vi "DBL Variant or Array Variant to Array.vi"(8 "error in (no error)":errorcluster, 11 "value":variant) -> (0 "error out":errorcluster, 3 "Array":dbl[](array[numeric]))   [LabVIEW 2019, in "SMO.Control Experiment.lvclass"]
uses:
  SMO.Control Experiment.lvclass
  <vilib>/Utility/Data Type/NI_Data Type.lvlib
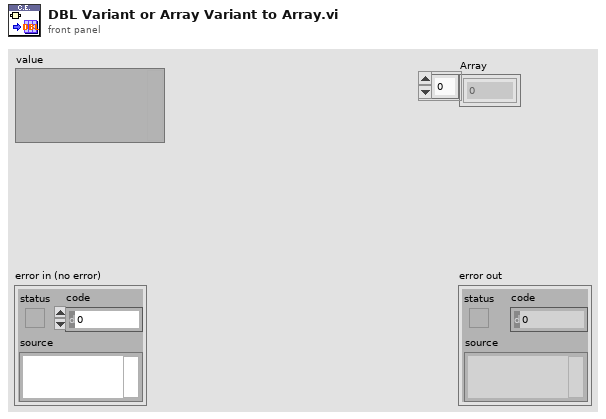
[diagram p1: front panel]
types:
  T1 = typedef "NI_Data Type.lvlib/Data Type.ctl" = enum8{"Invalid Type", "Void", "I8", "I16", "I32", "I64", "U8", "U16", "U32", "U64", "Single Float", "Double Float", "Extended Float", "Single Complex", "Double Complex", "Extended Complex", "Enum U8", "Enum U16", "Enum U32", "Enum U64", "Single Float With Unit", "Double Float With Unit", "Extended Float With Unit", "Single Complex with Unit", "Double Complex with Unit", "Extended Complex with Unit", "Boolean", "String", "Path", "Picture", "Tag", "Array", "Cluster", "Variant", "LV Variant", "Waveform", "Timestamp", "Digital Waveform", "Digital Data", "ExpressData", "Refnum", "External Data", "VI", "Poly VI", "LabVIEW Class Instance", "Fixed Point", "Set Collection", "Map Collection"}
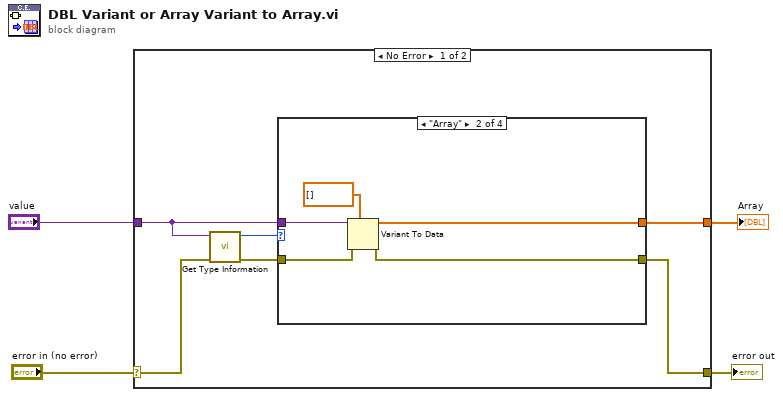
[diagram p0: block diagram]
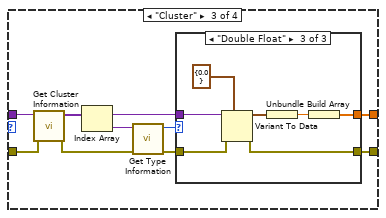
[diagram p3: hidden frame]
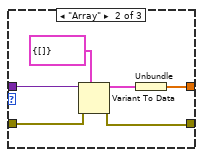
[diagram p5: hidden frame]
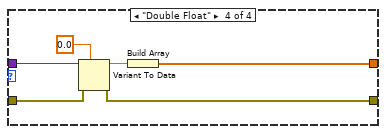
[diagram p6: hidden frame]
diagram:
  n1 = case shown="No Error" "error in (no error)" {
    selector: "error in (no error)" -> [w8 w46]
    tunnel: [w5 w46] -> w3
    tunnel: "value" -> [w9 _]
    tunnel: [w7 _] -> w1
    frame No Error {
      n2 = call <vilib>:"Get Type Information.vi"("error in (no error)"=w8, "variant"=w9) -> ("error out"=w6:errorcluster, "type"=w10:T1)  [unwired: 5 in, 3 out]
      n3 = case shown="\"Array\"" w10 {
        tunnel: [_ w15 w19 w41] -> w7
        tunnel: w9 -> [_ w14 w17 w44]
        tunnel: w6 -> [w11 w13 w25 w43]
        tunnel: [w11 w12 w18 w40] -> w5
        frame Default {
        }
        frame "Array" {
          n4 = Variant To Data(error in=w13, type=dbl[] [], Variant=w14) -> (data=w15:dbl[], error out=w12:errorcluster)
        }
        frame "Cluster" {
          n5 = call <vilib>:"Get Cluster Information.vi"("error in (no error)"=w25, "variant"=w17) -> ("error out"=w23:errorcluster, "cluster elements"=w24:variant[])  [unwired: 8 in]
          n6 = Index Array(array=w24) -> (element=w22:variant)  [unwired: 1 in]
          n7 = call <vilib>:"Get Type Information.vi"("error in (no error)"=w23, "variant"=w22) -> ("error out"=w20:errorcluster, "type"=w21:T1)  [unwired: 5 in, 3 out]
          n8 = case shown="\"Double Float\"" w21 {
            tunnel: [_ w27 w36] -> w19
            tunnel: w17 -> [_ w31 w38]
            tunnel: w20 -> [w26 w30 w37]
            tunnel: [w26 w29 w35] -> w18
            frame Default {
            }
            frame "Array" {
              n9 = Variant To Data(error in=w30, type=cluster{dbl[]} {[]}, Variant=w31) -> (data=w32:cluster{dbl[]}, error out=w29:errorcluster)
              n10 = Unbundle(w32) -> (w27:dbl[])
            }
            frame "Double Float" {
              n11 = Variant To Data(error in=w37, type=cluster{dbl} {0.0}, Variant=w38) -> (data=w39:cluster{dbl}, error out=w35:errorcluster)
              n12 = Unbundle(w39) -> (w33:dbl)
              n13 = Build Array(w33) -> (w36:dbl[])
            }
          }
        }
        frame "Double Float" {
          n14 = Variant To Data(error in=w43, type=0.0, Variant=w44) -> (data=w45:dbl, error out=w40:errorcluster)
          n15 = Build Array(w45) -> (w41:dbl[])
        }
      }
    }
    frame Error {
    }
  }
  "error out" <- w3
  "Array" <- w1
